vi "CreateHistogramArray.vi"() -> (3 "Array":i32[](array[numeric]))   [LabVIEW 2017]
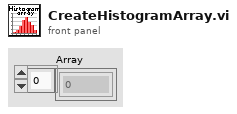
[diagram p1: front panel]
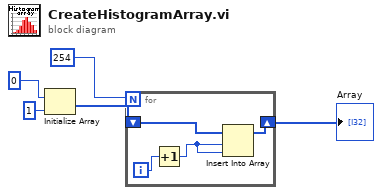
[diagram p0: block diagram]
diagram:
  n1 = Initialize Array(0, 1 ("dimension size")) -> (w3:i32[])
  n2 = for {
    N: 254 -> [_]
    shift-right: [w8] -> w1
    shift-left: w3 -> [w9]
    i -> [w7]
    n3 = Increment(x=w7) -> (x+1=w6:i32)
    n4 = Insert Into Array(array=w9, index=w6, new element=w6) -> (w8:i32[])
  }
  "Array" <- w1
